vi "CollectData.vi"(8 "error in (no error)":errorcluster, 11 "Master Device in":refnum<class "Master Device.lvclass">) -> (0 "error out":errorcluster, 3 "Master Device out":refnum<class "Master Device.lvclass">)   [LabVIEW 2013, in "Master Device.lvclass"]
uses:
  Master Device.lvclass
  Device/Device.lvclass
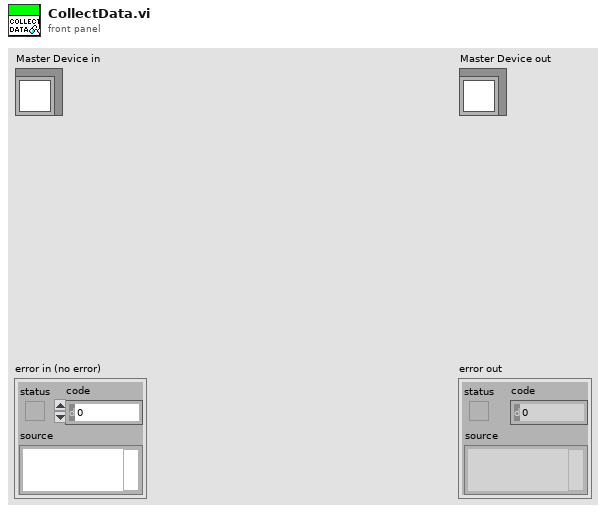
[diagram p1: front panel]
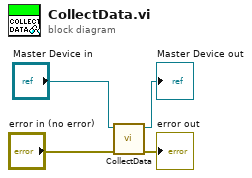
[diagram p0: block diagram]
diagram:
  n1 = call-parent "CollectData.vi"("error in (no error)"="error in (no error)", "Device in"="Master Device in") -> ("error out"=→"error out":errorcluster, "Device out"=→"Master Device out":refnum<class "Master Device.lvclass">)  [unwired: 8 in]
